vi "VMC.vi"() -> ()   [LabVIEW 2018]
doc: "PNA-X Example."
uses:
  PNA-X.lvlib
panel:
  out "VISA OUT":refnum<visa-resource-name>="GPIB1::16::INSTR"
  out "error out":errorcluster
  in  "error in (no error)":errorcluster
  out "XY Graph":cluster{"X-Axis":dbl[], "Data":dbl[]}(graph)
  in  "VISA IN":refnum<visa-resource-name>
  # "1. Select Instrument Source from the \"VISA IN\" drop down.\n2. Run vi"
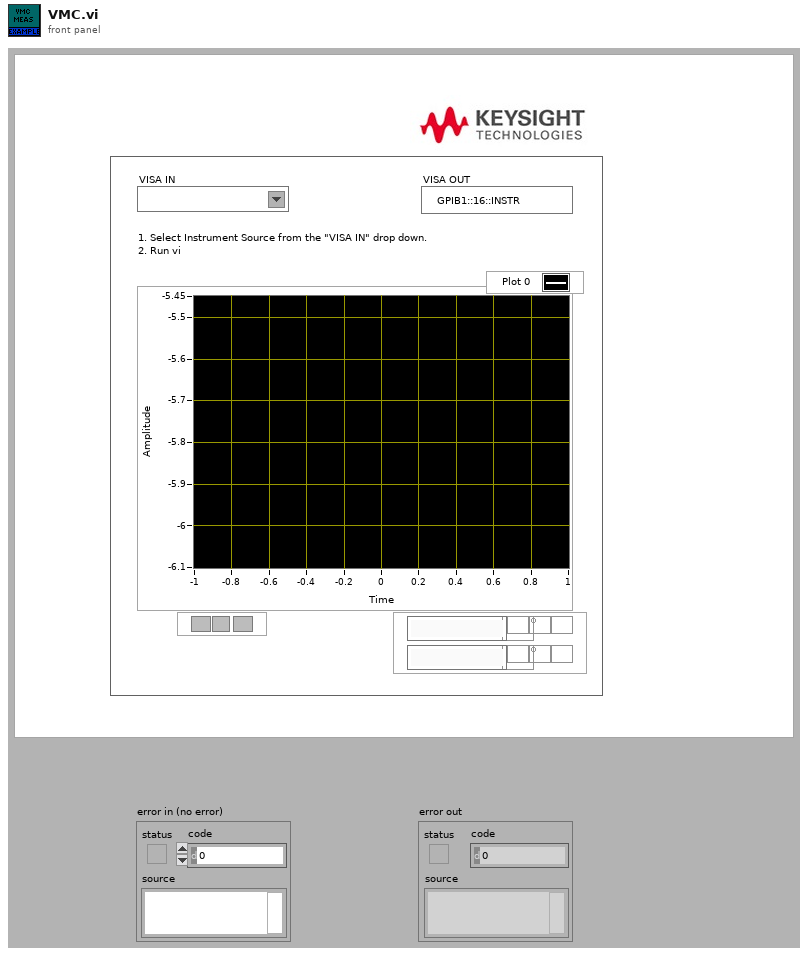
[diagram p1: front panel]
types:
  T1 = cluster{"Mixer file (*.mxr)":path, "Format":string, "Measurement":string, "OK Button":bool}
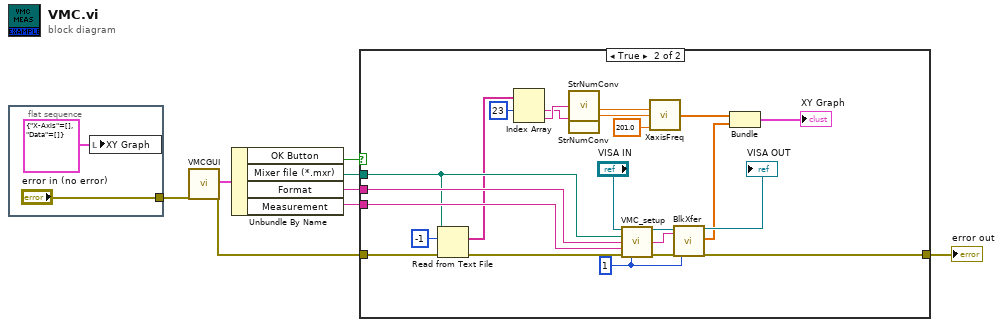
[diagram p0: block diagram]
diagram:
  n1 = flat-sequence {
    tunnel: ["error in (no error)"] -> w8
    frame #0 {
      n2 = local write "XY Graph"(cluster{"X-Axis":dbl[], "Data":dbl[]} {"X-Axis"=[], "Data"=[]} ("XY Graph")) -> ()
    }
  }
  n3 = call "VMCGUI.vi"("error in (no error)"=w8) -> ("output cluster"=w1:T1, "error out"=w5:errorcluster)  [unwired: 17 in]
  n4 = Unbundle By Name(w1) -> ("OK Button"=w6:bool, "Mixer file (*.mxr)"=w4:path, "Format"=w3:string, "Measurement"=w2:string)
  n5 = case shown="True" w6 {
    tunnel: [w11 w29] -> w7
    tunnel: w5 -> [w11 w21]
    tunnel: w4 -> [_ w18]
    tunnel: w3 -> [_ w23]
    tunnel: w2 -> [_ w22]
    frame False {
    }
    frame True {
      w31 = 1 ("Channel")
      n6 = Read from Text File(file (use dialog)=w18, count=-1, error in=w21) -> (text=w17:string[], error out=w20:errorcluster)  [unwired: 1 in, 2 out]
      n7 = Index Array(array=w17, index #1=23 ("index")) -> (element #1=w14:string, element #2=w15:string)  [unwired: 1 in]
      n8 = call "StrNumConv.vi"("Freq. String"=w15) -> ("Freq."=w13:dbl)  [unwired: 6 in]
      n9 = call "StrNumConv.vi"("Freq. String"=w14) -> ("Freq."=w12:dbl)  [unwired: 6 in]
      n10 = call "VMC_setup.vi"("PnaVisa"="VISA IN", "Mixer file (*.mxr)"=w18, "Format"=w23, "Measurement"=w22, "error in"=w20, "Channel"=w31) -> ("dup VISA session"=w33:refnum<visa-resource-name>, "FileName"=w30:string, "error out"=w32:errorcluster)  [unwired: 7 in]
      n11 = call "XaxisFreq.vi"("Start Frequency"=w13, "Stop Frequency"=w12, "Points"=201.0) -> ("X-Axis"=w26:dbl[])  [unwired: 12 in]
      n12 = call "BlkXfer.vi"("VISA IN"=w33, "FileName"=w30, "error in"=w32, "Channel"=w31) -> ("VISA Out"=→"VISA OUT":refnum<visa-resource-name>, "Data"=w27:dbl[], "error out"=w29:errorcluster)  [unwired: 13 in]
      n13 = Bundle("X-Axis"=w26, "Data"=w27) -> (→"XY Graph":cluster{"X-Axis":dbl[], "Data":dbl[]})  [unwired: 1 in]
    }
  }
  "error out" <- w7
